vi "Estimate Duty Cycle.vi"(3 "Nyquist Ratio":dbl=10.0, 4 "Rate (Hz)":dbl, 5 "Duration (ms)":dbl) -> (1 "Scan Rate (Hz)":dbl, 2 "Duty Cycle (%)":dbl)   [LabVIEW 2014]
doc: "Estimate the required duty cycle and sampling rate by provided signal characteristic. Nyquist oversampling rate is default to 10, e.g. for a 100Hz signal, it will estimate a 1kHz sampling rate is required."
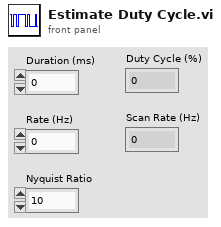
[diagram p1: front panel]
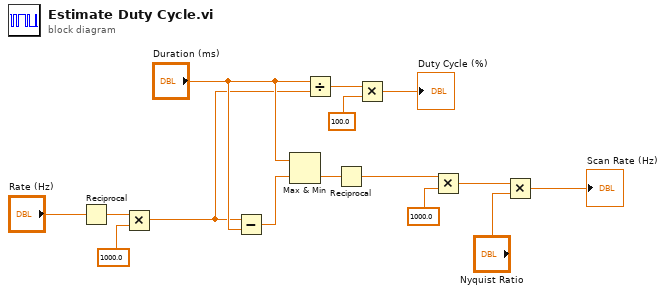
[diagram p0: block diagram]
diagram:
  n1 = Reciprocal(x="Rate (Hz)") -> (1/x=w14:dbl)
  n2 = Multiply(x=w14, y=1000.0) -> (x*y=w4:dbl)
  n3 = Subtract(x=w4, y="Duration (ms)") -> (x-y=w12:dbl)
  n4 = Max & Min(x="Duration (ms)", y=w12) -> (min(x,y)=w11:dbl)  [unwired: 1 out]
  n5 = Divide(x="Duration (ms)", y=w4) -> (x/y=w3:dbl)
  n6 = Reciprocal(x=w11) -> (1/x=w10:dbl)
  n7 = Multiply(x=w3, y=100.0) -> (x*y=→"Duty Cycle (%)":dbl)
  n8 = Multiply(x=w10, y=1000.0) -> (x*y=w8:dbl)
  n9 = Multiply(x=w8, y="Nyquist Ratio") -> (x*y=→"Scan Rate (Hz)":dbl)
